vi "Tail Deleted.vi"(3 "Snake in":refnum<class "Snake.lvclass">) -> (1 "Tail deleted":T1)   [LabVIEW 2021, in "Snake.lvclass"]
uses:
  Snake.lvclass
  Position.ctl
  Snake.lvclass/Snake.ctl
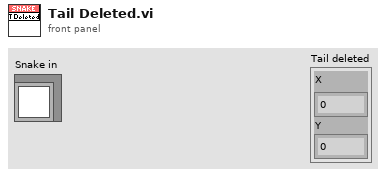
[diagram p1: front panel]
types:
  T1 = typedef "Position.ctl" = cluster{"X":u32, "Y":u32}
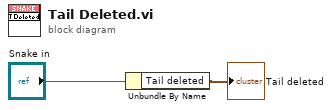
[diagram p0: block diagram]
diagram:
  n1 = Unbundle By Name("Snake in") -> ("Tail deleted"=→"Tail deleted":T1)
